vi "Read Status.vi"(8 "error in (no error)":errorcluster, 11 "SciShutt in":refnum<class "SciShutt.lvclass">) -> (0 "error out":errorcluster, 2 "Status":bool, 3 "SciShutt out":refnum<class "SciShutt.lvclass">)   [LabVIEW 2016, in "SciShutt.lvclass"]
uses:
  SciShutt.lvclass
  BiStable/BiStableShutter.lvclass
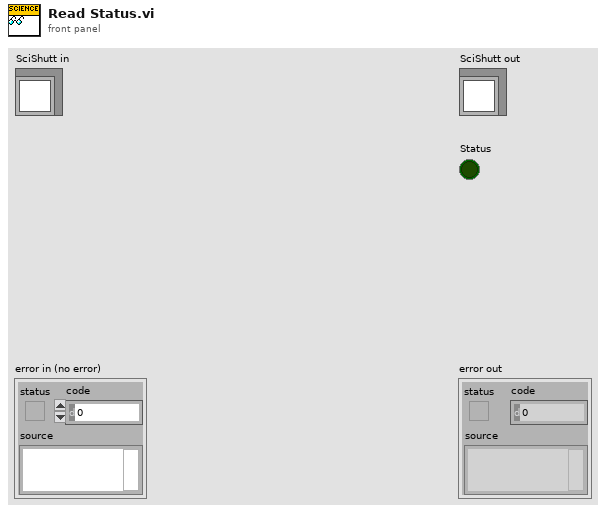
[diagram p1: front panel]
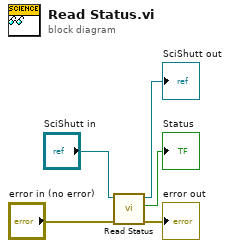
[diagram p0: block diagram]
diagram:
  n1 = call-parent "Read Status.vi"("error in (no error)"="error in (no error)", "Shutter in"="SciShutt in") -> ("error out"=→"error out":errorcluster, "Status"=→"Status":bool, "Shutter out"=→"SciShutt out":refnum<class "SciShutt.lvclass">)  [unwired: 7 in]
